vi "scan_equation.vi"(4 "Equation":string) -> (0 "Intercept":dbl, 1 "Angular Coefficient":dbl)   [LabVIEW 2021]
panel:
  out "b":string
  out "m":string
  out "after substring":string
  out "before substring":string
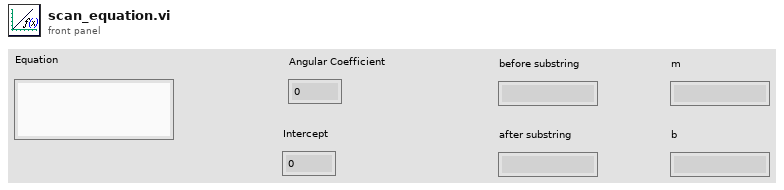
[diagram p1: front panel]
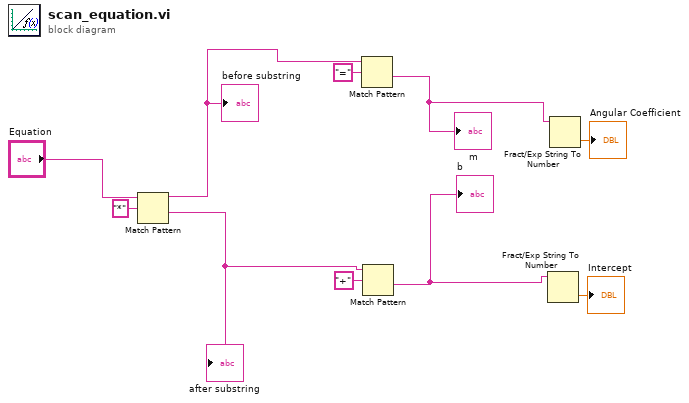
[diagram p0: block diagram]
diagram:
  n1 = Match Pattern(string="Equation", regular expression="*") -> (before substring=w8:string, after substring=w5:string)  [unwired: 1 in, 2 out]
  "before substring" <- w8
  "after substring" <- w5
  n2 = Match Pattern(string=w8, regular expression="=") -> (after substring=w4:string)  [unwired: 1 in, 3 out]
  "m" <- w4
  n3 = Match Pattern(string=w5, regular expression="+") -> (after substring=w3:string)  [unwired: 1 in, 3 out]
  "b" <- w3
  n4 = Fract/Exp String To Number(string=w3) -> (number=→"Intercept":dbl)  [unwired: 3 in, 1 out]
  n5 = Fract/Exp String To Number(string=w4) -> (number=→"Angular Coefficient":dbl)  [unwired: 3 in, 1 out]
